vi "write image data.vi"() -> ()   [LabVIEW 2020, in "sqlite3.lvlib"]
uses:
  sqlite3.lvlib
  sqlite/VIs/open v2.vi
  sqlite/VIs/prepare v2.vi
  sqlite/VIs/step.vi
  sqlite/VIs/column count.vi
  compound/Column.vi
  compound/Resolve Result Type.vi
  sqlite/VIs/finalize.vi
  sqlite/VIs/close v2.vi
  sqlite/subvi/Error Converter (ErrCode or Status).vi
  sqlite/VIs/column text.vi
  sqlite/VIs/column bytes.vi
  sqlite/VIs/column blob.vi
  utilities/MoveBlock.vi
  sqlite/VIs/column type.vi
  sqlite/VIs/errstr.vi
panel:
  in  "blob column name":string="image"
  in  "table name":string="blob"
  in  "database in":path=path "C:/labview/sqlite_dbManager/test database/blob.db"
  out "error out":errorcluster={"status"=TRUE, "code"=43, "source"="Write PNG File.vi"}
  in  "error in (no error)":errorcluster
  in  "Image file in":path=path "C:/labview/sqlite_dbManager/images/NLB_546989785EDR_D0622810TRAV00581M_-br2.jpg"
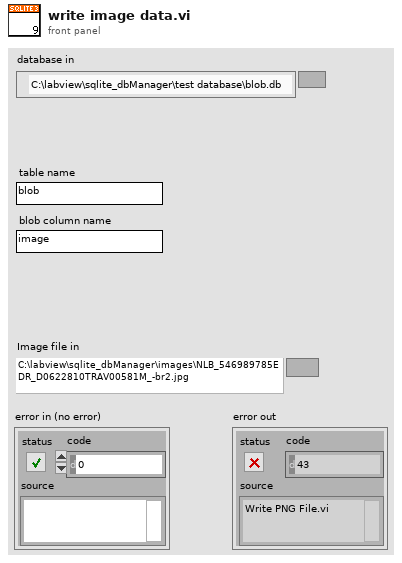
[diagram p1: front panel]
types:
  T1 = typedef "imagedata.ctl" = cluster{"image type":i32, "image depth":i32, "image":u8[], "mask":u8[], "colors":u32[], "Rectangle":cluster{"left":i16, "top":i16, "right":i16, "bottom":i16}}
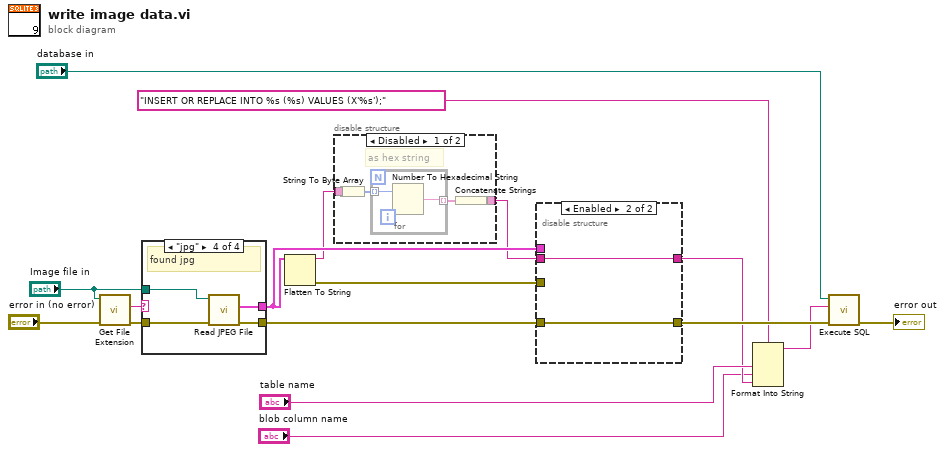
[diagram p0: block diagram]
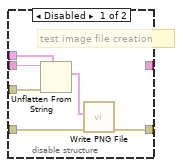
[diagram p3: hidden frame]
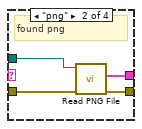
[diagram p5: hidden frame]
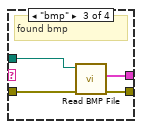
[diagram p6: hidden frame]
diagram:
  n1 = call <vilib>:"Get File Extension.vi"("error in (no error)"="error in (no error)", "file"="Image file in") -> ("error out"=w14:errorcluster, "lowercase file extension"=w16:string)  [unwired: 5 in, 3 out]
  n2 = case shown="\"jpg\"" w16 {
    tunnel: "Image file in" -> [_ w22 w26 w30]
    tunnel: [_ w21 w25 w29] -> w11
    tunnel: w14 -> [w18 w20 w23 w28]
    tunnel: [w18 w19 w24 w27] -> w13
    frame "False", Default {
      # "unsupported type"
    }
    frame "png" {
      # "found png"
      n3 = call <vilib>:"Read PNG File.vi"("error in (no error)"=w20, "path to PNG file"=w22) -> ("error out"=w19:errorcluster, "image data"=w21:T1)  [unwired: 7 in, 1 out]
    }
    frame "bmp" {
      # "found bmp"
      n4 = call <vilib>:"Read BMP File.vi"("error in (no error)"=w23, "path to BMP file"=w26) -> ("error out"=w24:errorcluster, "image data"=w25:T1)  [unwired: 7 in, 1 out]
    }
    frame "jpg" {
      # "found jpg"
      n5 = call <vilib>:"Read JPEG File.vi"("error in (no error)"=w28, "path to JPEG file"=w30) -> ("error out"=w27:errorcluster, "image data"=w29:T1)  [unwired: 7 in, 1 out]
    }
  }
  n6 = Flatten To String(anything=w11) -> (data string=w2:string, error out=w12:errorcluster)  [unwired: 3 in, 1 out]
  n7 = disable-structure shown="Disabled" {
    disable-tunnel: w2 -> [w32 w37]
    disable-tunnel: [w31 w37] -> w1
    frame Disabled {
      # "as hex string"
      n8 = String To Byte Array(string=w32) -> (unsigned byte array=w34:u8[])
      n9 = for {
        tunnel: w34 -> [w36] mode=indexing
        tunnel: [w35] -> w33 mode=indexing
        n10 = Number To Hexadecimal String(2:w36) -> (0:w35:string)  [unwired: 1 in]
      }
      n11 = Concatenate Strings(w33) -> (w31:string)
    }
    frame Enabled {
      # "as binary string"
    }
  }
  n12 = disable-structure shown="Enabled" {
    disable-tunnel: w13 -> [w43 w44]
    disable-tunnel: [w42 w44] -> w9
    disable-tunnel: w1 -> [w41 w45]
    disable-tunnel: w12 -> [w40 _]
    disable-tunnel: w11 -> [w38 _]
    disable-tunnel: [_ w45] -> w5
    frame Disabled {
      # "test image file creation"
      n13 = Unflatten From String(type=w38, binary string=w41, error in (no error)=w40) -> (value=w39:T1)  [unwired: 2 in, 2 out]
      n14 = call <vilib>:"Write PNG File.vi"("error in (no error)"=w43, "image data"=w39) -> ("error out"=w42:errorcluster)  [unwired: 8 in, 1 out]
    }
    frame Enabled {
    }
  }
  n15 = Format Into String(format string="INSERT OR REPLACE INTO %s (%s) VALUES (X'%s');", "table name", "blob column name", w5) -> (resulting string=w3:string)  [unwired: 2 in, 1 out]
  n16 = call "Execute SQL.vi"("error in (no error)"=w9, "sql (string)"=w3, "database in"="database in") -> ("error out"=→"error out":errorcluster)  [unwired: 7 in, 1 out]
